vi "byte_to_parameters.vi"(8 "error in (no error)":errorcluster, 10 "DeviceParam":u8[](array[numeric]), 11 "UV-VIS_AVANTES in":refnum<class "UV-VIS_AVANTES.lvclass">) -> (0 "error out":errorcluster, 2 "parameters cluster":T1, 3 "UV-VIS_AVANTES out":refnum<class "UV-VIS_AVANTES.lvclass">)   [LabVIEW 2015, in "UV-VIS_AVANTES.lvclass"]
uses:
  UV-VIS_AVANTES.lvclass
  def_parameters.ctl
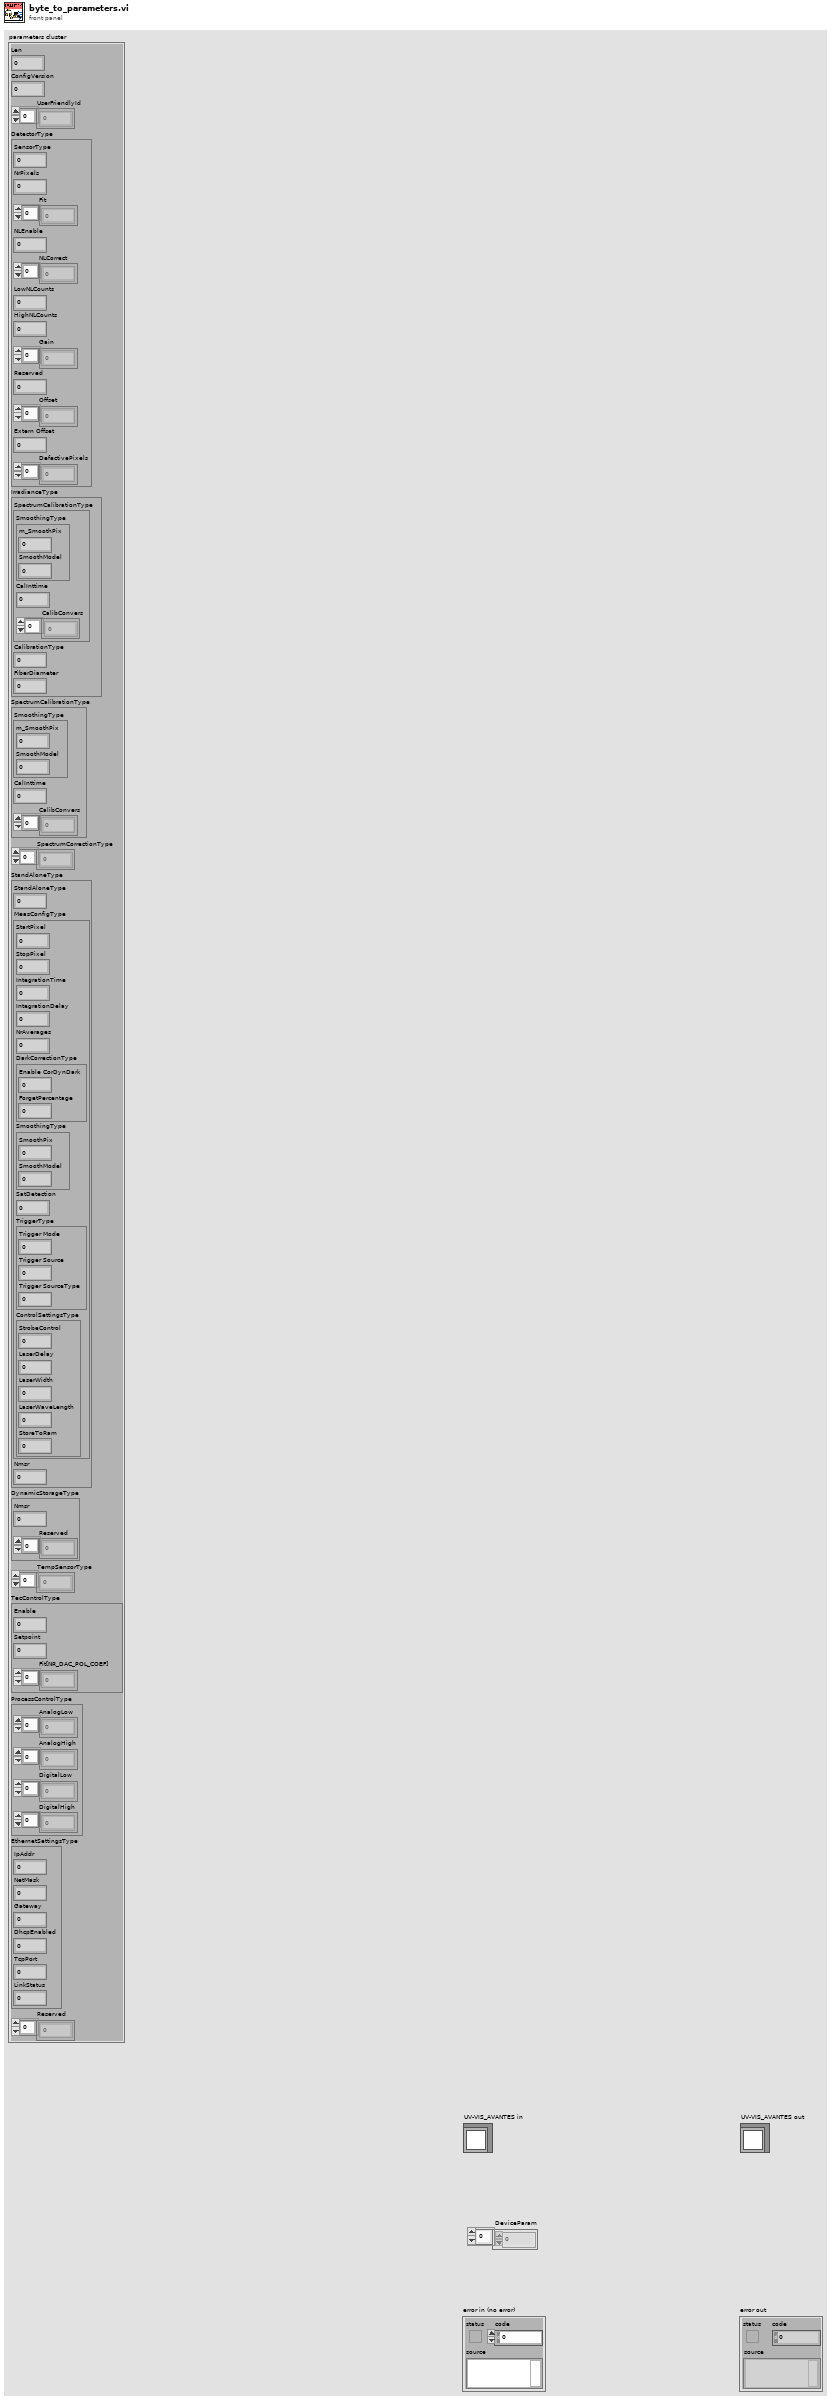
[diagram p1: front panel]
types:
  T1 = typedef "def_parameters.ctl" = cluster{"Len":u16, "ConfigVersion":u16, "UserFriendlyId":u8[], "DetectorType":cluster{"SensorType":u8, "NrPixels":u16, "Fit":sgl[], "NLEnable":u8, "NLCorrect":dbl[], "LowNLCounts":dbl, "HighNLCounts":dbl, "Gain":sgl[], "Reserved":sgl, "Offset":sgl[], "Extern Offset":sgl, "DefectivePixels":u16[]}, "IrradianceType":cluster{"SpectrumCalibrationType":cluster{"SmoothingType":cluster{"m_SmoothPix":u16, "SmoothModel":u8}, "CalInttime":sgl, "CalibConvers":sgl[]}, "CalibrationType":u8, "FiberDiameter":i32}, "SpectrumCalibrationType":cluster{"SmoothingType":cluster{"m_SmoothPix":u16, "SmoothModel":u8}, "CalInttime":sgl, "CalibConvers":sgl[]}, "SpectrumCorrectionType":sgl[], "StandAloneType":cluster{"StandAloneType":u8, "MeasConfigType":cluster{"StartPixel":u16, "StopPixel":u16, "IntegrationTime":sgl, "IntegrationDelay":u32, "NrAverages":u32, "DarkCorrectionType":cluster{"Enable CorDynDark":u8, "ForgetPercentage":u8}, "SmoothingType":cluster{"SmoothPix":u16, "SmoothModel":u8}, "SatDetection":u8, "TriggerType":cluster{"Trigger Mode":u8, "Trigger Source":u8, "Trigger SourceType":u8}, "ControlSettingsType":cluster{"StrobeControl":u16, "LaserDelay":u32, "LaserWidth":u32, "LaserWaveLength":sgl, "StoreToRam":u16}}, "Nmsr":i16}, "DynamicStorageType":cluster{"Nmsr":i32, "Reserved":u8[]}, "TempSensorType":sgl[], "TecControlType":cluster{"Enable":u8, "Setpoint":sgl, "Fit[NR_DAC_POL_COEF]":sgl[]}, "ProcessControlType":cluster{"AnalogLow":sgl[], "AnalogHigh":sgl[], "DigitalLow":sgl[], "DigitalHigh":sgl[]}, "EthernetSettingsType":cluster{"IpAddr":u32, "NetMask":u32, "Gateway":u32, "DhcpEnabled":u8, "TcpPort":u16, "LinkStatus":u8}, "Reserved":u8[]}
  T2 = cluster{u8, u16, sgl[], u8, dbl[], dbl, dbl, sgl[], sgl, sgl[], sgl, u16[]}
  T3 = cluster{u16, u16, sgl, u32, u32, cluster{u8, u8}, cluster{u16, u8}, u8, cluster{u8, u8, u8}, cluster{u16, u32, u32, sgl, u16}}
  T4 = cluster{cluster{cluster{u16, u8}, sgl, sgl[]}, u8, i32}
  T5 = cluster{u8, cluster{u16, u16, sgl, u32, u32, cluster{u8, u8}, cluster{u16, u8}, u8, cluster{u8, u8, u8}, cluster{u16, u32, u32, sgl, u16}}, i16}
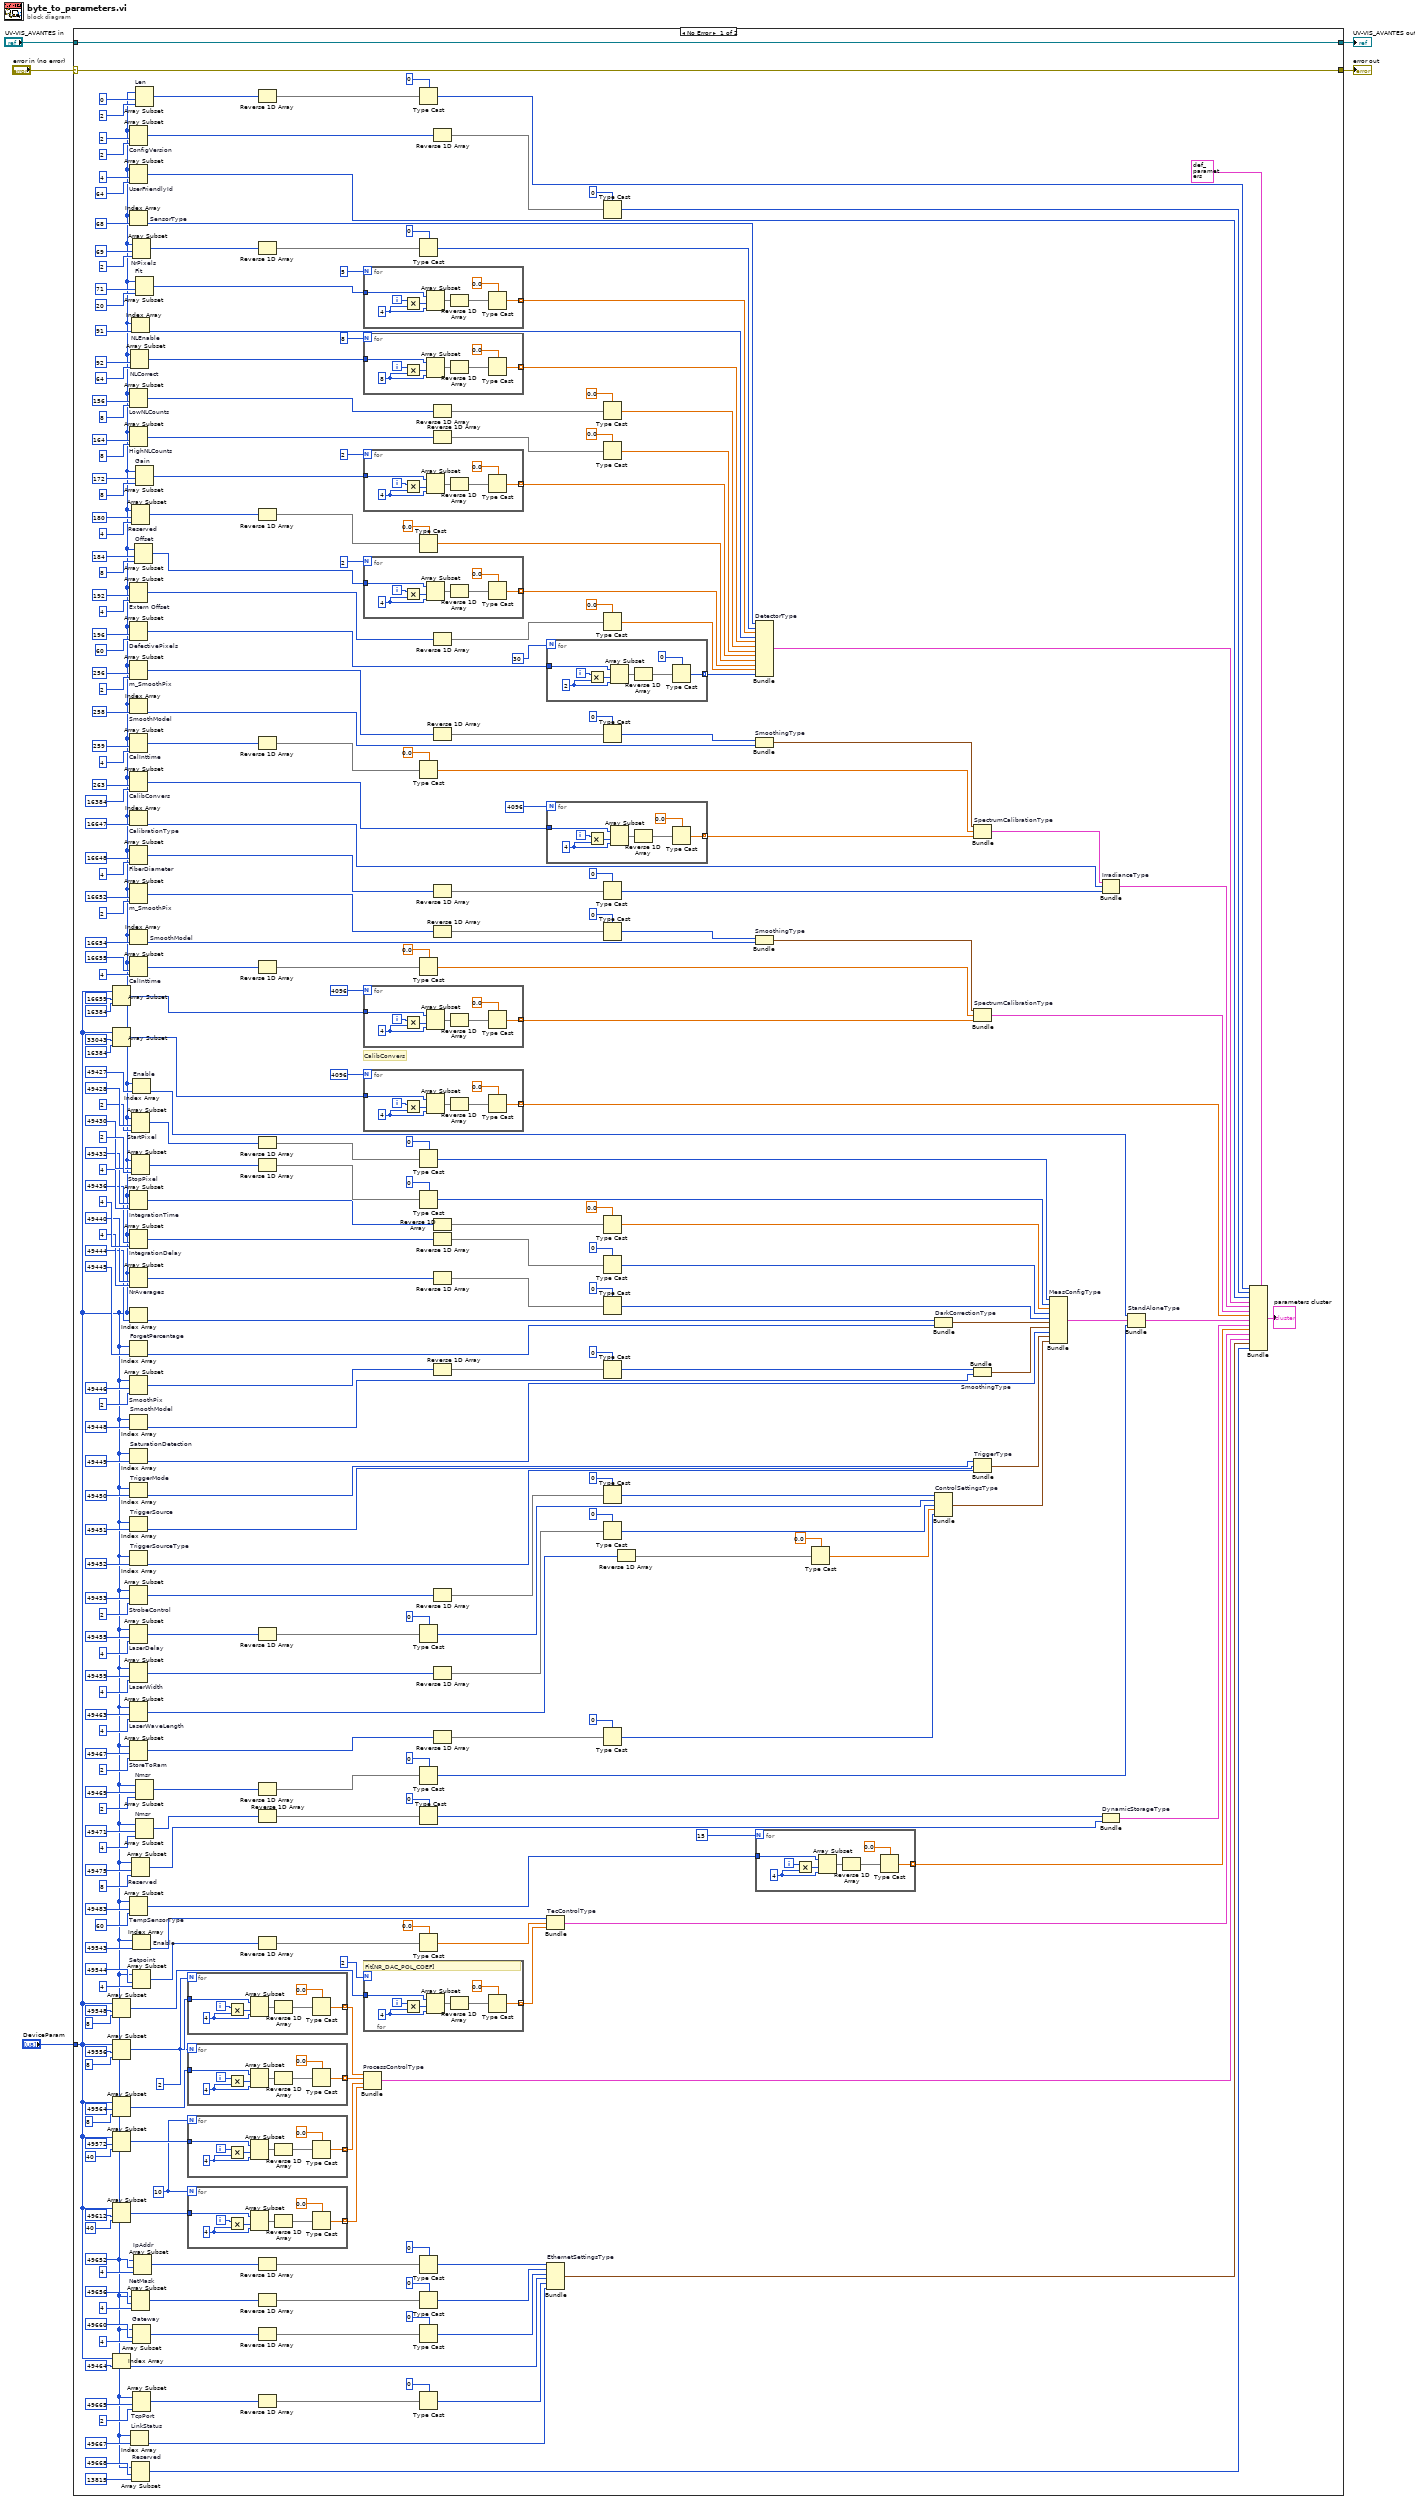
[diagram p0: block diagram]
diagram:
  n1 = case shown="No Error" "error in (no error)" {
    selector: "error in (no error)" -> [w10 w429]
    tunnel: "UV-VIS_AVANTES in" -> [w9 w428]
    tunnel: [w10 w429] -> w3
    tunnel: [w9 w428] -> w2
    tunnel: "DeviceParam" -> [w6 _]
    frame No Error {
      w8 = 10
      w7 = 2
      # "CalibConvers"
      n2 = Array Subset(array=w6, index=16659, length=16384) -> (w90:u8[])
      n3 = Array Subset(array=w6, index=33043, length=16384) -> (w91:u8[])
      n4 = Array Subset(array=w6, index=49548, length=8) -> (w73:u8[])
      n5 = Array Subset(array=w6, index=49556, length=8) -> (w68:u8[])
      n6 = Array Subset(array=w6, index=49564, length=8) -> (w65:u8[])
      n7 = Array Subset(array=w6, index=49572, length=40) -> (w62:u8[])
      n8 = Array Subset(array=w6, index=49612, length=40) -> (w59:u8[])
      n9 = Index Array(array=w6, index=49464 ("length")) -> (element=w20:u8)
      n10 = Array Subset "ConfigVersion"(array=w6, index=2, length=2) -> (w306:u8[])
      n11 = Array Subset "UserFriendlyId"(array=w6, index=4, length=64) -> (w139:u8[])
      n12 = Index Array "SensorType"(array=w6, index=68 ("length")) -> (element=w138:u8)
      n13 = Array Subset "LowNLCounts"(array=w6, index=156, length=8) -> (w288:u8[])
      n14 = Array Subset "HighNLCounts"(array=w6, index=164, length=8) -> (w285:u8[])
      n15 = Array Subset "Extern Offset"(array=w6, index=192, length=4) -> (w268:u8[])
      n16 = Array Subset "DefectivePixels"(array=w6, index=196, length=60) -> (w123:u8[])
      n17 = Array Subset "m_SmoothPix"(array=w6, index=256, length=2) -> (w259:u8[])
      n18 = Index Array "SmoothModel"(array=w6, index=258 ("length")) -> (element=w120:u8)
      n19 = Array Subset "CalInttime"(array=w6, index=259, length=4) -> (w255:u8[])
      n20 = Array Subset "CalibConvers"(array=w6, index=263, length=16384) -> (w118:u8[])
      n21 = Index Array "CalibrationType"(array=w6, index=16647 ("length")) -> (element=w116:u8)
      n22 = Array Subset "FiberDiameter"(array=w6, index=16648, length=4) -> (w246:u8[])
      n23 = Array Subset "m_SmoothPix"(array=w6, index=16652, length=2) -> (w233:u8[])
      n24 = Index Array "SmoothModel"(array=w6, index=16654 ("length")) -> (element=w112:u8)
      n25 = Array Subset "CalInttime"(array=w6, index=16655, length=4) -> (w236:u8[])
      n26 = Array Subset "IntegrationTime"(array=w6, index=49432, length=4) -> (w216:u8[])
      n27 = Array Subset "IntegrationDelay"(array=w6, index=49436, length=4) -> (w207:u8[])
      n28 = Array Subset "NrAverages"(array=w6, index=49440, length=4) -> (w204:u8[])
      n29 = Index Array "Index Array"(array=w6, index=49444 ("length")) -> (element=w99:u8)
      n30 = Index Array "ForgetPercentage"(array=w6, index=49445 ("length")) -> (element=w98:u8)
      n31 = Array Subset "SmoothPix"(array=w6, index=49446, length=2) -> (w198:u8[])
      n32 = Index Array "SmoothModel"(array=w6, index=49448 ("length")) -> (element=w96:u8)
      n33 = Index Array "SaturationDetection"(array=w6, index=49449 ("length")) -> (element=w95:u8)
      n34 = Index Array "TriggerMode"(array=w6, index=49450 ("length")) -> (element=w94:u8)
      n35 = Index Array "TriggerSource"(array=w6, index=49451 ("length")) -> (element=w93:u8)
      n36 = Index Array "TriggerSourceType"(array=w6, index=49452 ("length")) -> (element=w92:u8)
      n37 = Array Subset "StrobeControl"(array=w6, index=49453, length=2) -> (w186:u8[])
      n38 = Array Subset "LaserDelay"(array=w6, index=49455, length=4) -> (w183:u8[])
      n39 = Array Subset "LaserWidth"(array=w6, index=49459, length=4) -> (w176:u8[])
      n40 = Array Subset "LaserWaveLength"(array=w6, index=49463, length=4) -> (w173:u8[])
      n41 = Array Subset "StoreToRam"(array=w6, index=49467, length=2) -> (w166:u8[])
      n42 = Array Subset "TempSensorType"(array=w6, index=49483, length=60) -> (w83:u8[])
      n43 = Array Subset "NLCorrect"(array=w6, index=92, length=64) -> (w132:u8[])
      n44 = Index Array "LinkStatus"(array=w6, index=49667 ("length")) -> (element=w18:u8)
      n45 = Index Array "NLEnable"(array=w6, index=91 ("length")) -> (element=w134:u8)
      n46 = Array Subset "Reserved"(array=w6, index=180, length=4) -> (w276:u8[])
      n47 = Array Subset "StartPixel"(array=w6, index=49428, length=2) -> (w224:u8[])
      n48 = Array Subset "StopPixel"(array=w6, index=49430, length=2) -> (w219:u8[])
      n49 = Array Subset "Reserved"(array=w6, index=49475, length=8) -> (w82:u8[])
      n50 = Array Subset "NetMask"(array=w6, index=49656 ("length"), length=4) -> (w39:u8[])
      n51 = Array Subset "Reserved"(array=w6, index=49668, length=13815) -> (w17:u8[])
      n52 = Array Subset "Setpoint"(array=w6, index=49544, length=4) -> (w76:u8[])
      n53 = Array Subset "Gateway"(array=w6, index=49660 ("length"), length=4) -> (w34:u8[])
      n54 = Array Subset "TcpPort"(array=w6, index=49665 ("length"), length=2) -> (w26:u8[])
      n55 = Array Subset "NrPixels"(array=w6, index=69, length=2) -> (w302:u8[])
      n56 = Index Array "Enable"(array=w6, index=49427 ("length")) -> (element=w105:u8)
      n57 = Index Array "Enable"(array=w6, index=49543 ("length")) -> (element=w80:u8)
      n58 = Array Subset "IpAddr"(array=w6, index=49652 ("length"), length=4) -> (w44:u8[])
      n59 = Array Subset "Offset"(array=w6, index=184, length=8) -> (w125:u8[])
      n60 = Array Subset "Len"(array=w6, index=0, length=2) -> (w307:u8[])
      n61 = Array Subset "Fit"(array=w6, index=71, length=20) -> (w135:u8[])
      n62 = Array Subset "Gain"(array=w6, index=172, length=8) -> (w128:u8[])
      n63 = Array Subset "Nmsr"(array=w6, index=49469, length=2) -> (w161:u8[])
      n64 = Array Subset "Nmsr"(array=w6, index=49471 ("length"), length=4) -> (w51:u8[])
      n65 = for {
        N: w7 -> [_]
        tunnel: w68 -> [w344]
        tunnel: [w342] -> w56 mode=indexing
        i -> [w345]
        w346 = 4 ("length")
        n66 = Multiply(x=w345, y=w346) -> (x*y=w347:i32)
        n67 = Array Subset(array=w344, index=w347, length=w346) -> (w340:u8[])
        n68 = Reverse 1D Array(array=w340) -> (reversed array=w341:u8[])
        n69 = Type Cast(type=sgl 0.0, x=w341) -> (*(type *) &x=w342:sgl)
      }
      n70 = for {
        N: w7 -> [_]
        tunnel: w65 -> [w336]
        tunnel: [w334] -> w55 mode=indexing
        i -> [w337]
        w338 = 4 ("length")
        n71 = Multiply(x=w337, y=w338) -> (x*y=w339:i32)
        n72 = Array Subset(array=w336, index=w339, length=w338) -> (w332:u8[])
        n73 = Reverse 1D Array(array=w332) -> (reversed array=w333:u8[])
        n74 = Type Cast(type=sgl 0.0, x=w333) -> (*(type *) &x=w334:sgl)
      }
      n75 = for {
        N: w8 -> [_]
        tunnel: w62 -> [w328]
        tunnel: [w326] -> w54 mode=indexing
        i -> [w329]
        w330 = 4 ("length")
        n76 = Multiply(x=w329, y=w330) -> (x*y=w331:i32)
        n77 = Array Subset(array=w328, index=w331, length=w330) -> (w324:u8[])
        n78 = Reverse 1D Array(array=w324) -> (reversed array=w325:u8[])
        n79 = Type Cast(type=sgl 0.0, x=w325) -> (*(type *) &x=w326:sgl)
      }
      n80 = for {
        N: w8 -> [_]
        tunnel: w59 -> [w320]
        tunnel: [w318] -> w53 mode=indexing
        i -> [w321]
        w322 = 4 ("length")
        n81 = Multiply(x=w321, y=w322) -> (x*y=w323:i32)
        n82 = Array Subset(array=w320, index=w323, length=w322) -> (w316:u8[])
        n83 = Reverse 1D Array(array=w316) -> (reversed array=w317:u8[])
        n84 = Type Cast(type=sgl 0.0, x=w317) -> (*(type *) &x=w318:sgl)
      }
      n85 = Reverse 1D Array(array=w307) -> (reversed array=w150:u8[])
      n86 = Reverse 1D Array(array=w302) -> (reversed array=w303:u8[])
      n87 = Reverse 1D Array(array=w276) -> (reversed array=w275:u8[])
      n88 = Reverse 1D Array(array=w255) -> (reversed array=w256:u8[])
      n89 = Reverse 1D Array(array=w236) -> (reversed array=w235:u8[])
      n90 = Reverse 1D Array(array=w224) -> (reversed array=w225:u8[])
      n91 = Reverse 1D Array(array=w219) -> (reversed array=w218:u8[])
      n92 = Reverse 1D Array(array=w183) -> (reversed array=w184:u8[])
      n93 = Reverse 1D Array(array=w161) -> (reversed array=w160:u8[])
      n94 = Reverse 1D Array(array=w51) -> (reversed array=w52:u8[])
      n95 = Reverse 1D Array(array=w76) -> (reversed array=w75:u8[])
      n96 = Reverse 1D Array(array=w44) -> (reversed array=w45:u8[])
      n97 = Reverse 1D Array(array=w39) -> (reversed array=w40:u8[])
      n98 = Reverse 1D Array(array=w34) -> (reversed array=w35:u8[])
      n99 = Reverse 1D Array(array=w26) -> (reversed array=w27:u8[])
      n100 = for {
        N: 5 -> [_]
        tunnel: w135 -> [w424]
        tunnel: [w422] -> w136 mode=indexing
        i -> [w425]
        w426 = 4 ("length")
        n101 = Multiply(x=w425, y=w426) -> (x*y=w427:i32)
        n102 = Array Subset(array=w424, index=w427, length=w426) -> (w421:u8[])
        n103 = Reverse 1D Array(array=w421) -> (reversed array=w420:u8[])
        n104 = Type Cast(type=sgl 0.0, x=w420) -> (*(type *) &x=w422:sgl)
      }
      n105 = for {
        N: 8 -> [_]
        tunnel: w132 -> [w416]
        tunnel: [w414] -> w133 mode=indexing
        i -> [w417]
        w418 = 8 ("length")
        n106 = Multiply(x=w417, y=w418) -> (x*y=w419:i32)
        n107 = Array Subset(array=w416, index=w419, length=w418) -> (w413:u8[])
        n108 = Reverse 1D Array(array=w413) -> (reversed array=w412:u8[])
        n109 = Type Cast(type=0.0, x=w412) -> (*(type *) &x=w414:dbl)
      }
      n110 = for {
        N: 2 -> [_]
        tunnel: w128 -> [w408]
        tunnel: [w406] -> w129 mode=indexing
        i -> [w409]
        w410 = 4 ("length")
        n111 = Multiply(x=w409, y=w410) -> (x*y=w411:i32)
        n112 = Array Subset(array=w408, index=w411, length=w410) -> (w405:u8[])
        n113 = Reverse 1D Array(array=w405) -> (reversed array=w404:u8[])
        n114 = Type Cast(type=sgl 0.0, x=w404) -> (*(type *) &x=w406:sgl)
      }
      n115 = for {
        N: 2 -> [_]
        tunnel: w125 -> [w400]
        tunnel: [w398] -> w126 mode=indexing
        i -> [w401]
        w402 = 4 ("length")
        n116 = Multiply(x=w401, y=w402) -> (x*y=w403:i32)
        n117 = Array Subset(array=w400, index=w403, length=w402) -> (w397:u8[])
        n118 = Reverse 1D Array(array=w397) -> (reversed array=w396:u8[])
        n119 = Type Cast(type=sgl 0.0, x=w396) -> (*(type *) &x=w398:sgl)
      }
      n120 = for {
        N: 4096 -> [_]
        tunnel: w90 -> [w376]
        tunnel: [w374] -> w110 mode=indexing
        i -> [w377]
        w378 = 4 ("length")
        n121 = Multiply(x=w377, y=w378) -> (x*y=w379:i32)
        n122 = Array Subset(array=w376, index=w379, length=w378) -> (w373:u8[])
        n123 = Reverse 1D Array(array=w373) -> (reversed array=w372:u8[])
        n124 = Type Cast(type=sgl 0.0, x=w372) -> (*(type *) &x=w374:sgl)
      }
      n125 = for {
        N: 4096 -> [_]
        tunnel: w91 -> [w368]
        tunnel: [w366] -> w107 mode=indexing
        i -> [w369]
        w370 = 4 ("length")
        n126 = Multiply(x=w369, y=w370) -> (x*y=w371:i32)
        n127 = Array Subset(array=w368, index=w371, length=w370) -> (w365:u8[])
        n128 = Reverse 1D Array(array=w365) -> (reversed array=w364:u8[])
        n129 = Type Cast(type=sgl 0.0, x=w364) -> (*(type *) &x=w366:sgl)
      }
      n130 = for {
        N: 2 -> [_]
        tunnel: w73 -> [w352]
        tunnel: [w350] -> w69 mode=indexing
        i -> [w353]
        w354 = 4 ("length")
        # "Fit[NR_DAC_POL_COEF]"
        n131 = Multiply(x=w353, y=w354) -> (x*y=w355:i32)
        n132 = Array Subset(array=w352, index=w355, length=w354) -> (w348:u8[])
        n133 = Reverse 1D Array(array=w348) -> (reversed array=w349:u8[])
        n134 = Type Cast(type=sgl 0.0, x=w349) -> (*(type *) &x=w350:sgl)
      }
      n135 = Bundle "ProcessControlType"(w56, w55, w54, w53) -> (w15:cluster{sgl[], sgl[], sgl[], sgl[]})  [unwired: 1 in]
      n136 = Type Cast(type=u16 0, x=w150) -> (*(type *) &x=w141:u16)
      n137 = Type Cast(type=u16 0, x=w303) -> (*(type *) &x=w137:u16)
      n138 = Type Cast(type=sgl 0.0, x=w275) -> (*(type *) &x=w127:sgl)
      n139 = Type Cast(type=sgl 0.0, x=w256) -> (*(type *) &x=w119:sgl)
      n140 = Type Cast(type=sgl 0.0, x=w235) -> (*(type *) &x=w111:sgl)
      n141 = Type Cast(type=u16 0, x=w225) -> (*(type *) &x=w104:u16)
      n142 = Type Cast(type=u16 0, x=w218) -> (*(type *) &x=w103:u16)
      n143 = Type Cast(type=u32 0, x=w184) -> (*(type *) &x=w88:u32)
      n144 = Type Cast(type=i16 0, x=w160) -> (*(type *) &x=w84:i16)
      n145 = Type Cast(type=u32 0, x=w52) -> (*(type *) &x=w48:u32)
      n146 = Type Cast(type=sgl 0.0, x=w75) -> (*(type *) &x=w74:sgl)
      n147 = Type Cast(type=u32 0, x=w45) -> (*(type *) &x=w30:u32)
      n148 = Type Cast(type=u32 0, x=w40) -> (*(type *) &x=w29:u32)
      n149 = Type Cast(type=u32 0, x=w35) -> (*(type *) &x=w28:u32)
      n150 = Type Cast(type=u16 0, x=w27) -> (*(type *) &x=w19:u16)
      n151 = Reverse 1D Array(array=w306) -> (reversed array=w305:u8[])
      n152 = Reverse 1D Array(array=w288) -> (reversed array=w287:u8[])
      n153 = Reverse 1D Array(array=w285) -> (reversed array=w286:u8[])
      n154 = Reverse 1D Array(array=w268) -> (reversed array=w269:u8[])
      n155 = Reverse 1D Array(array=w259) -> (reversed array=w258:u8[])
      n156 = Reverse 1D Array(array=w246) -> (reversed array=w247:u8[])
      n157 = Reverse 1D Array(array=w233) -> (reversed array=w151:u8[])
      n158 = Reverse 1D Array(array=w216) -> (reversed array=w217:u8[])
      n159 = Reverse 1D Array(array=w207) -> (reversed array=w206:u8[])
      n160 = Reverse 1D Array(array=w204) -> (reversed array=w205:u8[])
      n161 = Reverse 1D Array(array=w198) -> (reversed array=w199:u8[])
      n162 = Reverse 1D Array(array=w186) -> (reversed array=w185:u8[])
      n163 = Reverse 1D Array(array=w176) -> (reversed array=w175:u8[])
      n164 = Reverse 1D Array(array=w166) -> (reversed array=w167:u8[])
      n165 = for {
        N: 30 -> [_]
        tunnel: w123 -> [w392]
        tunnel: [w390] -> w122 mode=indexing
        i -> [w393]
        w394 = 2 ("length")
        n166 = Multiply(x=w393, y=w394) -> (x*y=w395:i32)
        n167 = Array Subset(array=w392, index=w395, length=w394) -> (w389:u8[])
        n168 = Reverse 1D Array(array=w389) -> (reversed array=w388:u8[])
        n169 = Type Cast(type=u16 0, x=w388) -> (*(type *) &x=w390:u16)
      }
      n170 = for {
        N: 4096 -> [_]
        tunnel: w118 -> [w384]
        tunnel: [w382] -> w117 mode=indexing
        i -> [w385]
        w386 = 4 ("length")
        n171 = Multiply(x=w385, y=w386) -> (x*y=w387:i32)
        n172 = Array Subset(array=w384, index=w387, length=w386) -> (w381:u8[])
        n173 = Reverse 1D Array(array=w381) -> (reversed array=w380:u8[])
        n174 = Type Cast(type=sgl 0.0, x=w380) -> (*(type *) &x=w382:sgl)
      }
      n175 = Bundle "TecControlType"(w80, w74, w69) -> (w14:cluster{u8, sgl, sgl[]})  [unwired: 1 in]
      n176 = Bundle "EthernetSettingsType"(w30, w29, w28, w20, w19, w18) -> (w16:cluster{u32, u32, u32, u8, u16, u8})  [unwired: 1 in]
      n177 = Type Cast(type=u16 0, x=w305) -> (*(type *) &x=w140:u16)
      n178 = Type Cast(type=0.0, x=w287) -> (*(type *) &x=w131:dbl)
      n179 = Type Cast(type=0.0, x=w286) -> (*(type *) &x=w130:dbl)
      n180 = Type Cast(type=sgl 0.0, x=w269) -> (*(type *) &x=w124:sgl)
      n181 = Type Cast(type=u16 0, x=w258) -> (*(type *) &x=w121:u16)
      n182 = Type Cast(type=0, x=w247) -> (*(type *) &x=w115:i32)
      n183 = Type Cast(type=u16 0, x=w151) -> (*(type *) &x=w113:u16)
      n184 = Type Cast(type=sgl 0.0, x=w217) -> (*(type *) &x=w102:sgl)
      n185 = Type Cast(type=u32 0, x=w206) -> (*(type *) &x=w101:u32)
      n186 = Type Cast(type=u32 0, x=w205) -> (*(type *) &x=w100:u32)
      n187 = Type Cast(type=u16 0, x=w199) -> (*(type *) &x=w97:u16)
      n188 = Type Cast(type=u16 0, x=w185) -> (*(type *) &x=w89:u16)
      n189 = Type Cast(type=u32 0, x=w175) -> (*(type *) &x=w87:u32)
      n190 = Type Cast(type=u16 0, x=w167) -> (*(type *) &x=w85:u16)
      n191 = Reverse 1D Array(array=w173) -> (reversed array=w174:u8[])
      n192 = Bundle "DetectorType"(w138, w137, w136, w134, w133, w131, w130, w129, w127, w126, w124, w122) -> (w149:T2)  [unwired: 1 in]
      n193 = Bundle "SmoothingType"(w121, w120) -> (w144:cluster{u16, u8})  [unwired: 1 in]
      n194 = Bundle "SmoothingType"(w113, w112) -> (w114:cluster{u16, u8})  [unwired: 1 in]
      n195 = for {
        N: 15 -> [_]
        tunnel: w83 -> [w360]
        tunnel: [w358] -> w13 mode=indexing
        i -> [w361]
        w362 = 4 ("length")
        n196 = Multiply(x=w361, y=w362) -> (x*y=w363:i32)
        n197 = Array Subset(array=w360, index=w363, length=w362) -> (w356:u8[])
        n198 = Reverse 1D Array(array=w356) -> (reversed array=w357:u8[])
        n199 = Type Cast(type=sgl 0.0, x=w357) -> (*(type *) &x=w358:sgl)
      }
      n200 = Type Cast(type=sgl 0.0, x=w174) -> (*(type *) &x=w86:sgl)
      n201 = Bundle "DarkCorrectionType"(w99, w98) -> (w145:cluster{u8, u8})  [unwired: 1 in]
      n202 = Bundle "ControlSettingsType"(w89, w88, w87, w86, w85) -> (w142:cluster{u16, u32, u32, sgl, u16})  [unwired: 1 in]
      n203 = Bundle "SpectrumCalibrationType"(w144, w119, w117) -> (w109:cluster{cluster{u16, u8}, sgl, sgl[]})  [unwired: 1 in]
      n204 = Bundle "SpectrumCalibrationType"(w114, w111, w110) -> (w108:cluster{cluster{u16, u8}, sgl, sgl[]})  [unwired: 1 in]
      n205 = Bundle "SmoothingType"(w97, w96) -> (w106:cluster{u16, u8})  [unwired: 1 in]
      n206 = Bundle "TriggerType"(w94, w93, w92) -> (w143:cluster{u8, u8, u8})  [unwired: 1 in]
      n207 = Bundle "MeasConfigType"(w104, w103, w102, w101, w100, w145, w106, w95, w143, w142) -> (w146:T3)  [unwired: 1 in]
      n208 = Bundle "IrradianceType"(w109, w116, w115) -> (w148:T4)  [unwired: 1 in]
      n209 = Bundle "DynamicStorageType"(w48, w82) -> (w12:cluster{u32, u8[]})  [unwired: 1 in]
      n210 = Bundle "StandAloneType"(w105, w146, w84) -> (w147:T5)  [unwired: 1 in]
      n211 = Bundle(cluster=T1 {"Len"=0, "ConfigVersion"=0, "UserFriendlyId"=[], "DetectorType"={"SensorType"=0, "NrPixels"=0, "Fit"=[], "NLEnable"=0, "NLCorrect"=[], "LowNLCounts"=0.0, "HighNLCounts"=0.0, "Gain"=[], "Reserved"=0.0, "Offset"=[], "Extern Offset"=0.0, "DefectivePixels"=[]}, "IrradianceType"={"SpectrumCalibrationType"={"SmoothingType"={"m_SmoothPix"=0, "SmoothModel"=0}, "CalInttime"=0.0, "CalibConvers"=[]}, "CalibrationType"=0, "FiberDiameter"=0}, "SpectrumCalibrationType"={"SmoothingType"={"m_SmoothPix"=0, "SmoothModel"=0}, "CalInttime"=0.0, "CalibConvers"=[]}, "SpectrumCorrectionType"=[], "StandAloneType"={"StandAloneType"=0, "MeasConfigType"={"StartPixel"=0, "StopPixel"=0, "IntegrationTime"=0.0, "IntegrationDelay"=0, "NrAverages"=0, "DarkCorrectionType"={"Enable CorDynDark"=0, "ForgetPercentage"=0}, "SmoothingType"={"SmoothPix"=0, "SmoothModel"=0}, "SatDetection"=0, "TriggerType"={"Trigger Mode"=0, "Trigger Source"=0, "Trigger SourceType"=0}, "ControlSettingsType"={"StrobeControl"=0, "LaserDelay"=0, "LaserWidth"=0, "LaserWaveLength"=0.0, "StoreToRam"=0}}, "Nmsr"=0}, "DynamicStorageType"={"Nmsr"=0, "Reserved"=[]}, "TempSensorType"=[], "TecControlType"={"Enable"=0, "Setpoint"=0.0, "Fit[NR_DAC_POL_COEF]"=[]}, "ProcessControlType"={"AnalogLow"=[], "AnalogHigh"=[], "DigitalLow"=[], "DigitalHigh"=[]}, "EthernetSettingsType"={"IpAddr"=0, "NetMask"=0, "Gateway"=0, "DhcpEnabled"=0, "TcpPort"=0, "LinkStatus"=0}, "Reserved"=[]} ("DeviceConfig"), "Len"=w141, "ConfigVersion"=w140, "UserFriendlyId"=w139, "DetectorType"=w149, "IrradianceType"=w148, "SpectrumCalibrationType"=w108, "SpectrumCorrectionType"=w107, "StandAloneType"=w147, "DynamicStorageType"=w12, "TempSensorType"=w13, "TecControlType"=w14, "ProcessControlType"=w15, "EthernetSettingsType"=w16, "Reserved"=w17) -> (→"parameters cluster":T1)
    }
    frame Error {
    }
  }
  "error out" <- w3
  "UV-VIS_AVANTES out" <- w2
